vi "Get 1D Array Double.vi"(5 "use temporary file? (F)":bool, 7 "data type of variable":dbl[](array[numeric]), 8 "error in":errorcluster, 10 "variable name":string, 11 "GOLPI ref. in":T1={"pipe handle"={"lv_proc.dll file path"=path "", "process instance handle"=[], "debug mode"=FALSE, "debug data"=[]}, "fast read timeout [ms]"=500, "fast read settle time [ms]"=10, "fast read to multiple [ms]"=1, "max elements per input line"=100, "slow read timeout [ms]"=5000, "stdin double format specifier"="%_16e", "max elements per stdout output column"=100, "console mode bitstream"=FALSE, "bitstream first read timeout [ms]"=1000, "bitstream read timeout [ms]"=50, "struct transfer possible"=FALSE, "matlab mode"=FALSE}) -> (0 "error out":errorcluster, 2 "value":dbl[](array[numeric]) format="%.2f", 3 "GOLPI ref. out":T1={"pipe handle"={"lv_proc.dll file path"=path "", "process instance handle"=[], "debug mode"=FALSE, "debug data"=[]}, "fast read timeout [ms]"=500, "fast read settle time [ms]"=10, "fast read to multiple [ms]"=1, "max elements per input line"=100, "slow read timeout [ms]"=5000, "stdin double format specifier"="%_16e", "max elements per stdout output column"=100, "console mode bitstream"=FALSE, "bitstream first read timeout [ms]"=1000, "bitstream read timeout [ms]"=50, "struct transfer possible"=FALSE, "matlab mode"=FALSE})   [LabVIEW 2020, in "GOLPI library.lvlib"]
doc: "Part of polymorph Get Variable.vi"
uses:
  GOLPI library.lvlib
  GOLPI reference Type Def.ctl
  Pipe Handle.ctl
  Bitstream Data Type.ctl
  Custom Error Codes Enum Type Def.vi
  LV Process library.lvlib
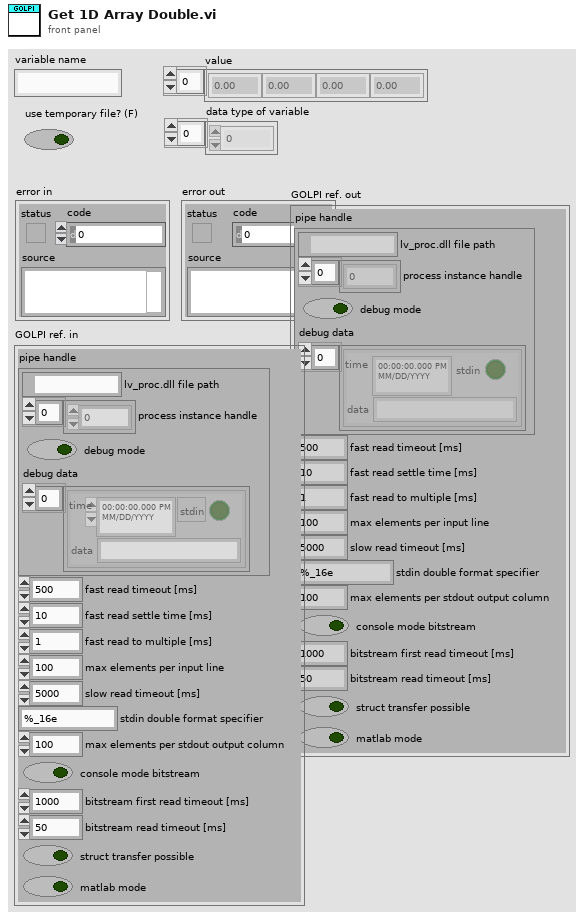
[diagram p1: front panel]
types:
  T1 = typedef "GOLPI library.lvlib/GOLPI reference Type Def.ctl" = cluster{"pipe handle":T2, "fast read timeout [ms]":u32, "fast read settle time [ms]":u32, "fast read to multiple [ms]":u32, "max elements per input line":u32, "slow read timeout [ms]":u32, "stdin double format specifier":string, "max elements per stdout output column":u32, "console mode bitstream":bool, "bitstream first read timeout [ms]":u32, "bitstream read timeout [ms]":u32, "struct transfer possible":bool, "matlab mode":bool}
  T2 = typedef "LV Process library.lvlib/Pipe Handle.ctl" = cluster{"lv_proc.dll file path":path, "process instance handle":u32[], "debug mode":bool, "debug data":cluster{"time":timestamp, "stdin":bool, "data":string}[]}
  T3 = typedef "GOLPI library.lvlib/Bitstream Data Type.ctl" = enum16{"dummy", "int", "uint", "float", "complex", "str", "real numeric"}
  T4 = typedef "GOLPI library.lvlib/Custom Error Codes Enum Type Def.vi" = enum16{"no error", "00 working directory PAR1 missing", "01 octave binary PAR1 missing", "02 octave report error PAR1", "03 empty output last cmd PAR1", "04 missing temporary file PAR1", "05 pwd PAR 1 not exist", "06 oct package not installed", "07 octave default binary missing", "10 var PAR1 not string, vect", "11 var PAR1 not num, scal, ~compl", "12 var PAR1 not num, scal, compl", "13 var PAR1 not num, vect, ~compl", "14 var PAR1 not num, vect, compl", "15 var PAR1 not num, mat, ~compl", "16 var PAR1 not num, mat, ~compl", "30 read timeout", "60 bitstream transport failed", "61 bitstream decode error PAR1", "62 bitstream cannot be set", "70 struct transfer not possible", "80 struct: cluster elem. PAR1 not implem.", "81 struct: structure field PAR1 not implem.", "82 struct: size mismatch of PAR1", "83 struct: type mismatch of PAR1", "98 internal error", "99 not finished", "90 Not supported in Matlab mode", "91 Matlab variable transfer error", "92 Matlab Script Error"}
  T5 = typedef "GOLPI library.lvlib/Bitstream Data.ctl" = cluster{"double":dbl[][], "cplx double":cdb[][], "int64":i64[][], "uint64":u64[][], "str":string[], "data type":T3}
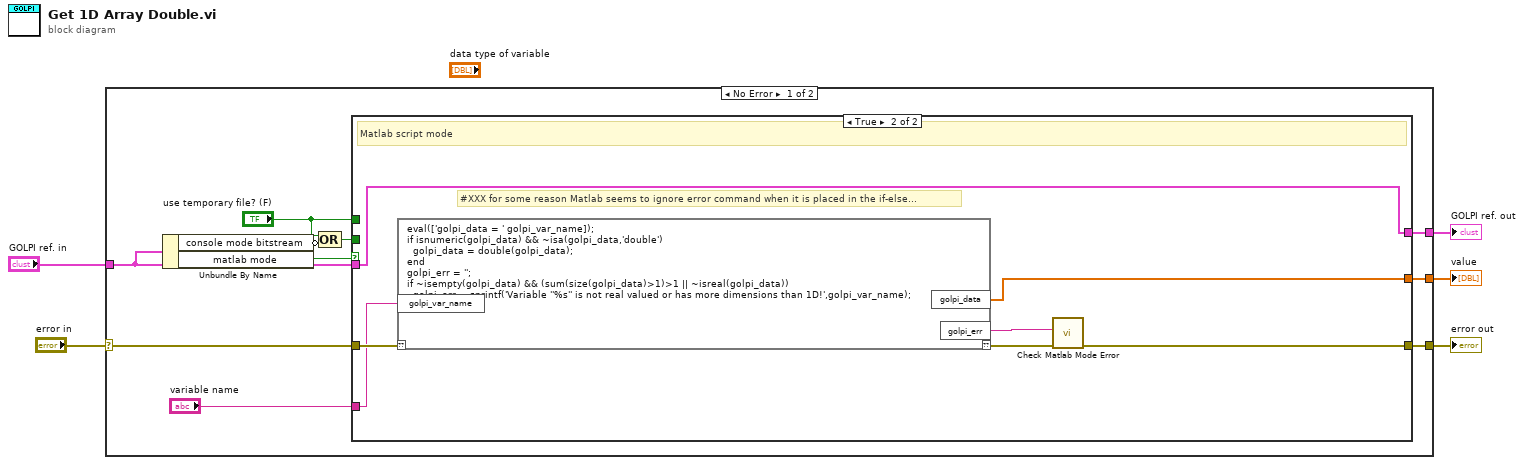
[diagram p0: block diagram]
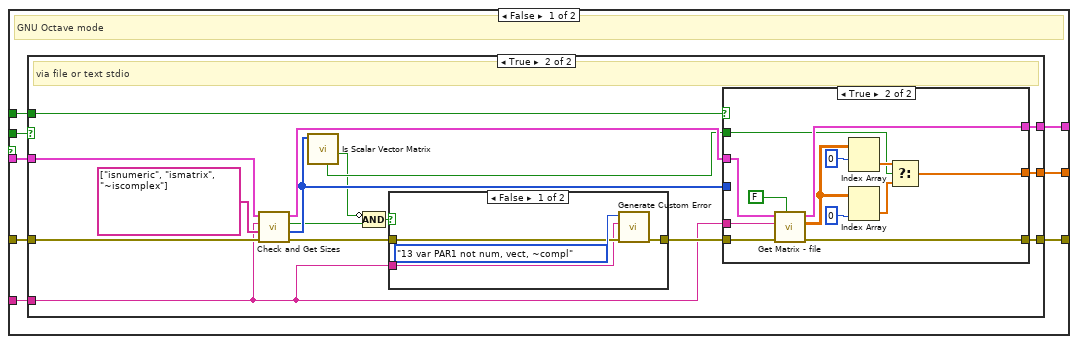
[diagram p2: hidden frame]
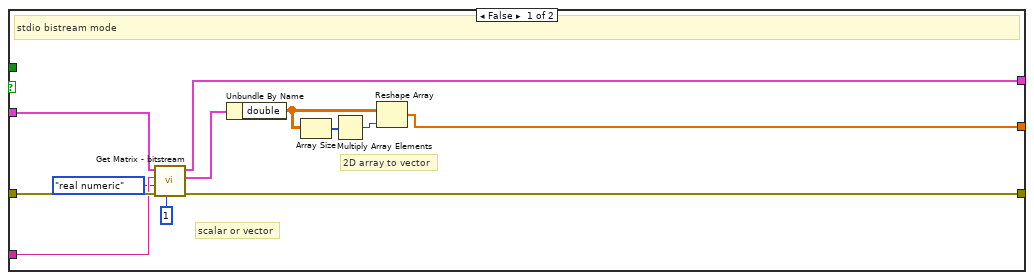
[diagram p3: hidden frame]
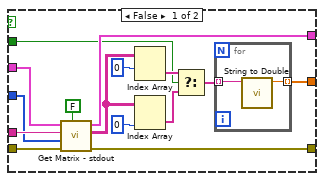
[diagram p4: hidden frame]
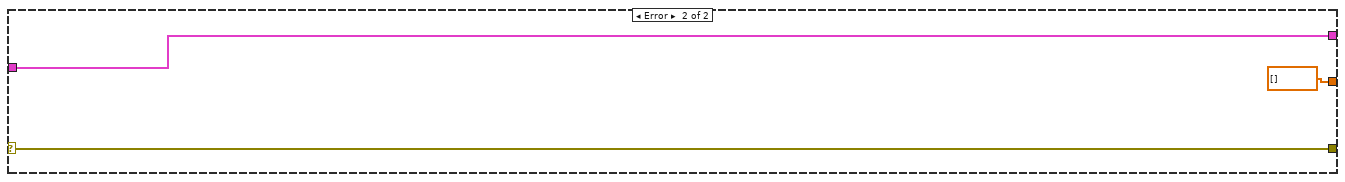
[diagram p6: hidden frame]
diagram:
  n1 = case shown="No Error" "error in" {
    selector: "error in" -> [w14 w96]
    tunnel: [w13 w96] -> w5
    tunnel: [w15 dbl[] [] ("value")] -> w3
    tunnel: "GOLPI ref. in" -> [w10 w94]
    tunnel: [w11 w94] -> w1
    frame No Error {
      n2 = Unbundle By Name(w10) -> ("console mode bitstream"=w9:bool, "matlab mode"=w6:bool)
      n3 = Compound Arithmetic op=OR("use temporary file? (F)", invert w9) -> (w7:bool)
      n4 = case shown="True" w6 {
        tunnel: [w23 w90] -> w15
        tunnel: w14 -> [w22 w93]
        tunnel: [w21 w88] -> w13
        tunnel: "variable name" -> [w20 w91]
        tunnel: [w19 w92] -> w11
        tunnel: w10 -> [w18 w92]
        tunnel: "use temporary file? (F)" -> [w17 _]
        tunnel: w7 -> [w16 _]
        frame False {
          # "GNU Octave mode"
          n5 = case shown="True" w16 {
            tunnel: [w24 w51] -> w23
            tunnel: w22 -> [w35 w50]
            tunnel: [w33 w45] -> w21
            tunnel: w20 -> [w32 w44]
            tunnel: w17 -> [_ w43]
            tunnel: w18 -> [w34 w42]
            tunnel: [w29 w41] -> w19
            frame False {
              # "2D array to vector"
              # "scalar or vector"
              # "stdio bistream mode"
              n6 = call "Get Matrix - bitstream.vi"("max dimensions (0: scalar)"=1, "error in (no error)"=w35, "data type"=Bitstream_Data_Type."real numeric", "variable name"=w32, "GOLPI ref. in"=w34) -> ("error out"=w33:errorcluster, "data"=w28:T5, "GOLPI ref. out"=w29:T1)  [unwired: 4 in]
              n7 = Unbundle By Name(w28) -> ("double"=w27:dbl[][])
              n8 = Array Size(array=w27) -> (size(s)=w26:i32[])
              n9 = Multiply Array Elements(1:w26) -> (0:w25:i32)
              n10 = Reshape Array(w27, w25) -> (w24:dbl[])
            }
            frame True {
              # "via file or text stdio"
              n11 = call "Check and Get Sizes.vi"("error in (no error)"=w50, "test commands"=string[] ["isnumeric", "ismatrix", "~iscomplex"], "variable name"=w44, "GOLPI ref. in"=w42) -> ("error out"=w49:errorcluster, "octave sizes"=w40:i32[], "all tests OK?"=w37:bool, "GOLPI ref. out"=w47:T1)  [unwired: 4 in]
              n12 = call "Is Scalar Vector Matrix.vi"("octave sizes"=w40) -> ("is matrix?"=w36:bool, "row vector?"=w39:bool)  [unwired: 5 in, 4 out]
              n13 = Compound Arithmetic op=AND(invert w36, w37) -> (w38:bool)
              n14 = case shown="False" w38 {
                tunnel: w49 -> [w84 w86]
                tunnel: [w83 w86] -> w46
                tunnel: w44 -> [w82 _]
                frame False {
                  n15 = call "Generate Custom Error.vi"("error in"=w84, "PAR1"=w82, "GOLPI error"=Custom_Error_Codes_Enum_Type_Def.vi."13 var PAR1 not num, vect, ~compl" ("Enum")) -> ("error out"=w83:errorcluster)  [unwired: 8 in]
                }
                frame True {
                }
              }
              n16 = case shown="True" w43 {
                tunnel: [w52 w74] -> w51
                tunnel: w47 -> [w59 w80]
                tunnel: [w55 w79] -> w41
                tunnel: w46 -> [w60 w77]
                tunnel: [w56 w76] -> w45
                tunnel: w44 -> [w58 w78]
                tunnel: w40 -> [w57 _]
                tunnel: w39 -> [w54 w69]
                frame False {
                  n17 = call "Get Matrix - stdout.vi"("is string?"=FALSE ("is string"), "error in (no error)"=w60, "octave sizes"=w57, "variable name"=w58, "GOLPI ref. in"=w59) -> ("error out"=w56:errorcluster, "array"=w61:string[][], "GOLPI ref. out"=w55:T1)  [unwired: 4 in]
                  n18 = Index Array(array=w61, index (row)=0) -> (element=w63:string[])  [unwired: 1 in]
                  n19 = Index Array(array=w61, index (col)=0 ("disabled index (col)")) -> (element=w62:string[])  [unwired: 1 in]
                  n20 = Select(t=w63, s=w54, f=w62) -> (s? t:f=w53:string[])
                  n21 = for {
                    tunnel: w53 -> [w68] mode=indexing
                    tunnel: [w67] -> w52 mode=indexing
                    n22 = call "String to Double.vi"("string"=w68) -> ("number"=w67:dbl)  [unwired: 10 in]
                  }
                }
                frame True {
                  n23 = call "Get Matrix - file.vi"("is string?"=FALSE ("is string"), "error in (no error)"=w77, "variable name"=w78, "GOLPI ref. in"=w80) -> ("error out"=w76:errorcluster, "double array"=w72:dbl[][], "GOLPI ref. out"=w79:T1)  [unwired: 3 in, 2 out]
                  n24 = Index Array(array=w72, index (row)=0) -> (element=w73:dbl[])  [unwired: 1 in]
                  n25 = Index Array(array=w72, index (col)=0 ("disabled index (col)")) -> (element=w75:dbl[])  [unwired: 1 in]
                  n26 = Select(t=w73, s=w69, f=w75) -> (s? t:f=w74:dbl[])
                }
              }
            }
          }
        }
        frame True {
          # "#XXX for some reason Matlab seems to ignore error command when it is placed in the if-else..."
          # "Matlab script mode"
          n27 = script code="eval(['golpi_data = ' golpi_var_name]);\nif isnumeric(golpi_data) && ~isa(golpi_data,'double')\n  golpi_data = double(golpi_data);\nend\ngolpi_err = '';\nif ~isempty(golpi_data) && (sum(size(golpi_data)>1)>1 || ~isreal(golpi_data))\n  golpi_err = sprintf('Variable ''%s'' is not real valued or has more dimensions than 1D!',golpi_var_name);\nend"("??"=w93, "golpi_var_name"=w91) -> ("??"=w89:errorcluster, "golpi_data"=w90:dbl[], "golpi_err"=w87:string)
          n28 = call "Check Matlab Mode Error.vi"("error in"=w89, "custom error string (empty)"=w87) -> ("error out"=w88:errorcluster)  [unwired: 9 in]
        }
      }
    }
    frame Error {
    }
  }
  "value" <- w3
  "error out" <- w5
  "GOLPI ref. out" <- w1
